vi "_TreeItem.Property.Set.Dictionary.Write.vi"(8 "error in (no error)":errorcluster, 11 "Dictionary":T1) -> (0 "error out":errorcluster, 3 "DictionaryProperty":refnum<k39>)   [LabVIEW 2027, in "Advanced System Definition.lvlib"]
uses:
  SysDef API/Advanced System Definition.lvlib
  _Types/Dictionary Item.ctl
  _Types/Property.Dictionary.ctl
  C:/NetCoreDLL/NationalInstruments.VeriStand.SystemStorage.dll
  NetCoreDLL/NationalInstruments.VeriStand.SystemStorage.dll
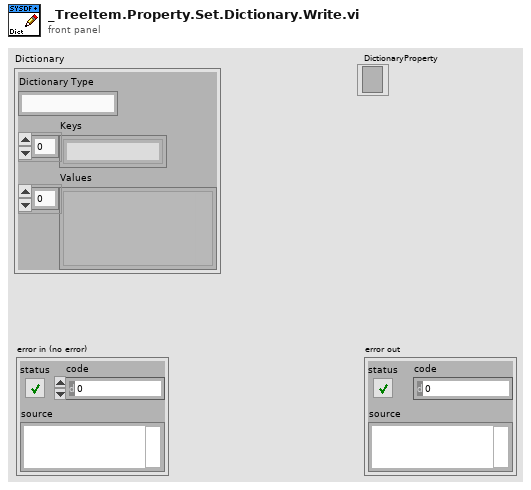
[diagram p1: front panel]
types:
  T1 = typedef "Advanced System Definition.lvlib/Property.Dictionary.ctl" = cluster{"Dictionary Type":string, "Keys":string[], "Values":variant[]}
  T2 = typedef "Advanced System Definition.lvlib/Dictionary Item.ctl" = cluster{"index":i32, "key":string, "value":variant}
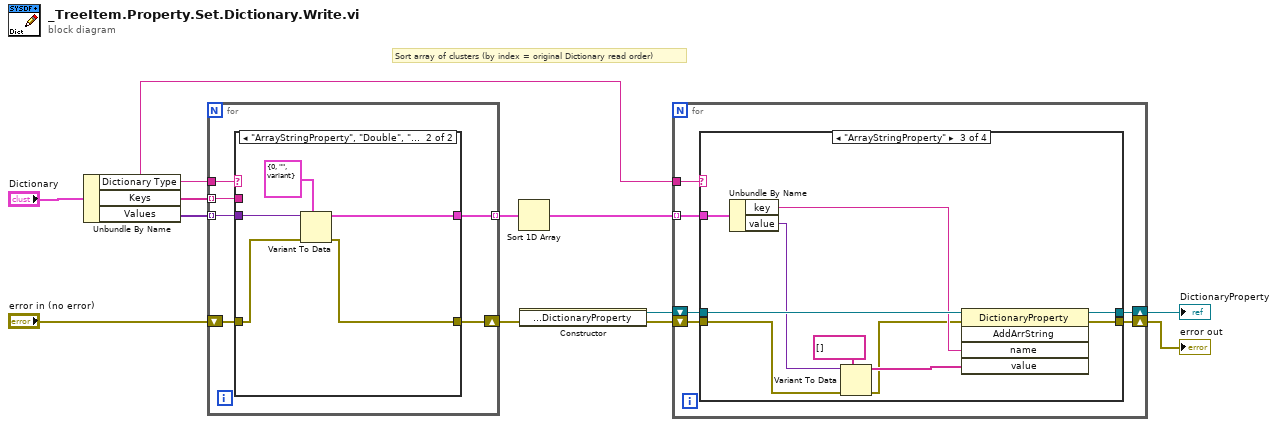
[diagram p0: block diagram]
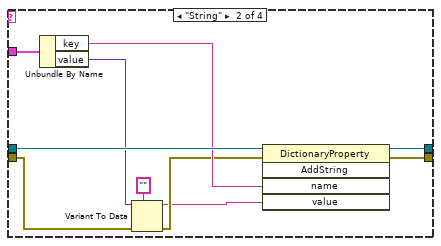
[diagram p3: hidden frame]
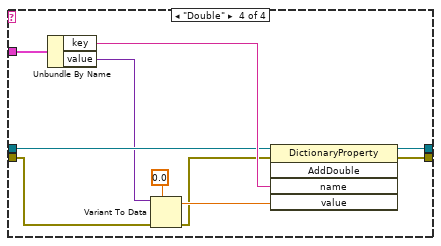
[diagram p4: hidden frame]
diagram:
  # "Sort array of clusters (by index = original Dictionary read order)"
  n1 = Unbundle By Name("Dictionary") -> ("Dictionary Type"=w9:string, "Keys"=w10:string[], "Values"=w11:variant[])
  n2 = for {
    tunnel: w9 -> [w18]
    tunnel: w11 -> [w17] mode=indexing
    tunnel: w10 -> [w16] mode=indexing
    shift-right: [w14] -> w4
    shift-left: "error in (no error)" -> [w15]
    tunnel: [w13] -> w6 mode=indexing
    n3 = case shown="\"ArrayStringProperty\", \"Double\", \"String\"" w18 {
      tunnel: w16 -> [_ _]
      tunnel: w17 -> [_ w24]
      tunnel: w15 -> [w19 w23]
      tunnel: [w19 w22] -> w14
      tunnel: [_ w21] -> w13
      frame Default {
      }
      frame "ArrayStringProperty", "Double", "String" {
        n4 = Variant To Data(error in=w23, type=T2 {"index"=0, "key"="", "value"=variant} ("Dictionary Item"), Variant=w24) -> (data=w21:T2, error out=w22:errorcluster)
      }
    }
  }
  n5 = Sort 1D Array(array=w6) -> (sorted array=w5:T2[])
  n6 = constructor class="DictionaryProperty"(error in=w4) -> (reference out=w2:refnum<k39>, error out=w3:errorcluster)  [unwired: 2 in, 1 out]
  n7 = for {
    shift-right: [w29] -> w8
    shift-left: w2 -> [w30]
    tunnel: w9 -> [w28]
    shift-right: [w26] -> w7
    shift-left: w3 -> [w27]
    tunnel: w5 -> [w25] mode=indexing
    n8 = case shown="\"ArrayStringProperty\"" w28 {
      tunnel: w30 -> [w32 w42 w52 w58]
      tunnel: [w32 w41 w51 w62] -> w29
      tunnel: w27 -> [w31 w35 w44 w54]
      tunnel: [w31 w40 w50 w61] -> w26
      tunnel: w25 -> [_ w39 w48 w59]
      frame Default {
      }
      frame "String" {
        n9 = Unbundle By Name(w39) -> ("key"=w38:string, "value"=w36:variant)
        n10 = Variant To Data(error in=w35, type="", Variant=w36) -> (data=w33:string, error out=w34:errorcluster)
        n11 = invoke class="DictionaryProperty" method="AddString"(reference=w42, error in=w34, "name"=w38, "value"=w33) -> (reference out=w41:refnum<k39>, error out=w40:errorcluster)  [unwired: 1 in, 3 out]
      }
      frame "ArrayStringProperty" {
        n12 = Unbundle By Name(w48) -> ("key"=w49:string, "value"=w46:variant)
        n13 = Variant To Data(error in=w44, type=string[] [], Variant=w46) -> (data=w45:string[], error out=w43:errorcluster)
        n14 = invoke class="DictionaryProperty" method="AddArrString"(reference=w52, error in=w43, "name"=w49, "value"=w45) -> (reference out=w51:refnum<k39>, error out=w50:errorcluster)  [unwired: 1 in, 3 out]
      }
      frame "Double" {
        n15 = Unbundle By Name(w59) -> ("key"=w60:string, "value"=w56:variant)
        n16 = Variant To Data(error in=w54, type=0.0, Variant=w56) -> (data=w55:dbl, error out=w53:errorcluster)
        n17 = invoke class="DictionaryProperty" method="AddDouble"(reference=w58, error in=w53, "name"=w60, "value"=w55) -> (reference out=w62:refnum<k39>, error out=w61:errorcluster)  [unwired: 1 in, 3 out]
      }
    }
  }
  "error out" <- w7
  "DictionaryProperty" <- w8
